vi "FindCommand+Contents.vi"(0 "Via file in":string) -> (2 "left":string, 3 "Contents":string, 4 "command":string, 5 "success":bool)   [LabVIEW 2012]
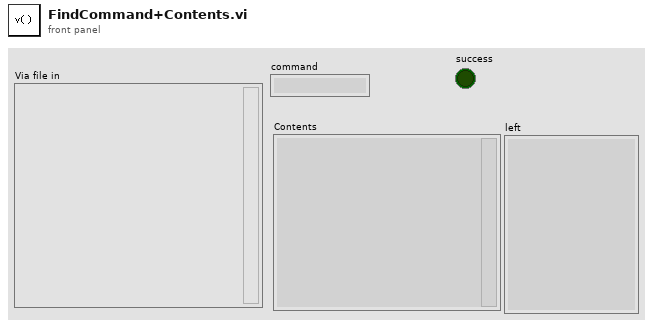
[diagram p1: front panel]
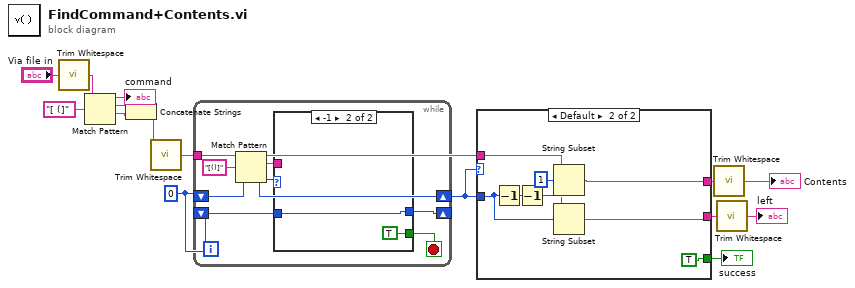
[diagram p0: block diagram]
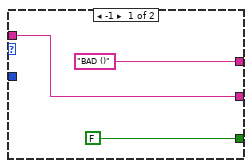
[diagram p2: hidden frame]
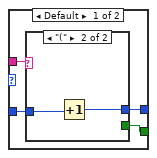
[diagram p3: hidden frame]
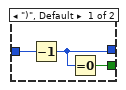
[diagram p4: hidden frame]
diagram:
  w9 = 0
  n1 = call <vilib>:"Trim Whitespace.vi"("string"="Via file in") -> ("trimmed string"=w4:string)  [unwired: 1 in]
  n2 = Match Pattern(string=w4, regular expression="[ (]") -> (before substring=→"command":string, match substring=w11:string, after substring=w12:string)  [unwired: 1 in, 1 out]
  n3 = Concatenate Strings(w11, w12) -> (w13:string)
  n4 = call <vilib>:"Trim Whitespace.vi"("string"=w13) -> ("trimmed string"=w14:string)  [unwired: 1 in]
  n5 = while {
    tunnel: w14 -> [w23]
    shift-right: [w18] -> w15
    shift-left: w9 -> [w19]
    shift-right: [w16] -> _
    shift-left: w9 -> [w17]
    stop <- w21 stop-if-true
    n6 = Match Pattern(string=w23, regular expression="[()]", offset (0)=w19) -> (match substring=w20:string, offset past match=w18:i32)  [unwired: 2 out]
    n7 = case shown="-1" w18 {
      tunnel: [w24 TRUE] -> w21
      tunnel: w20 -> [w27 _]
      tunnel: w17 -> [w26 w33]
      tunnel: [w25 w33] -> w16
      frame Default {
        n8 = case shown="\"(\"" w27 {
          tunnel: w26 -> [w30 w32]
          tunnel: [w29 w31] -> w25
          tunnel: [w28 _] -> w24
          frame ")", Default {
            n9 = Decrement(x=w30) -> (x-1=w29:i32)
            n10 = Equal To 0?(x=w29) -> (x = 0?=w28:bool)
          }
          frame "(" {
            n11 = Increment(x=w32) -> (x+1=w31:i32)
          }
        }
      }
      frame -1 {
      }
    }
  }
  n12 = case shown="Default" w15 {
    tunnel: w15 -> [_ w39]
    tunnel: ["BAD ()" ("trimmed string") w44] -> w10
    tunnel: w14 -> [w35 w41]
    tunnel: [FALSE TRUE] -> w5
    tunnel: [w35 w38] -> w2
    frame -1 {
    }
    frame Default {
      n13 = Decrement(x=w39) -> (x-1=w40:i32)
      n14 = Decrement(x=w40) -> (x-1=w42:i32)
      n15 = String Subset(string=w41, offset (0)=1, length (rest)=w42) -> (substring=w44:string)
      n16 = String Subset(string=w41, offset (0)=w39) -> (substring=w38:string)  [unwired: 1 in]
    }
  }
  "success" <- w5
  n17 = call <vilib>:"Trim Whitespace.vi"("string"=w10) -> ("trimmed string"=→"Contents":string)  [unwired: 1 in]
  n18 = call <vilib>:"Trim Whitespace.vi"("string"=w2) -> ("trimmed string"=→"left":string)  [unwired: 1 in]
